vi "Join HDC Bank2 DIO.vi"(5 "IN 7:6":fxp<+,2,2> format="%02b", 6 "IN 5":bool, 7 "IN 4:3":fxp<+,2,2> format="%02b", 8 "IN 0":bool, 9 "IN 2":bool, 10 "IN 1":bool) -> (2 "OUT 7:0":u8 format="%08b")   [LabVIEW 2017]
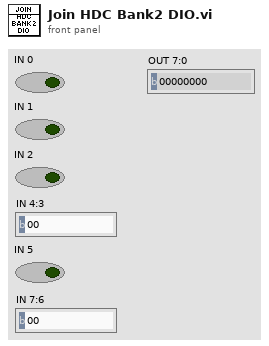
[diagram p1: front panel]
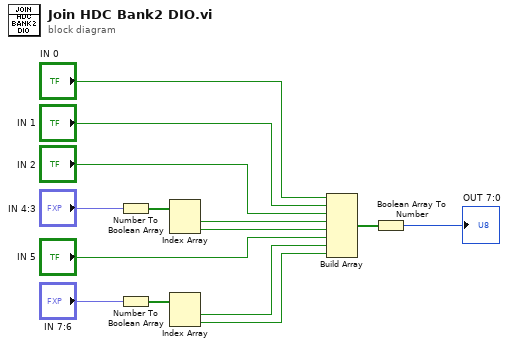
[diagram p0: block diagram]
diagram:
  n1 = Number To Boolean Array(number="IN 4:3") -> (Boolean array=w8:bool[])
  n2 = Number To Boolean Array(number="IN 7:6") -> (Boolean array=w13:bool[])
  n3 = Index Array(array=w8) -> (element #1=w3:bool, element #2=w2:bool)  [unwired: 2 in]
  n4 = Index Array(array=w13) -> (element #1=w11:bool, element #2=w10:bool)  [unwired: 2 in]
  n5 = Build Array("IN 0", "IN 1", "IN 2", w3, w2, "IN 5", w11, w10) -> (w9:bool[])
  n6 = Boolean Array To Number(Boolean array=w9) -> (number=→"OUT 7:0":u8)
